vi "LINX - Serial to TCP test.vi"() -> ()   [LabVIEW 2020]
uses:
  <vilib>/MakerHub/LINX/Private/Device/Type Defs/Wifi Config.ctl
  <vilib>/MakerHub/LINX/Private/Type Defs/WIFI Security Type.ctl
  <vilib>/MakerHub/LINX/Private/Device/Type Defs/TCP Config.ctl
  <vilib>/MakerHub/LINX/Public/Utilities/Open Serial.vi
  <vilib>/MakerHub/LINX/Public/Utilities/Open TCP.vi
  <vilib>/MakerHub/LINX/LMH-LINX.lvlib
  <vilib>/MakerHub/LINX/Private/Device/Device.lvlib
panel:
  out "LINX Device Config.TCP Configuration":T1
  in  "stop":bool
  in  "Wifi Configuration":T2={"SSID"="", "IP Address"="0.0.0.0", "Port"=44300, "WIFI Security Type"=enum."WPA2 Password", "Password"=""}
  in  "Serial Port":refnum<visa-resource-name>="N/A"
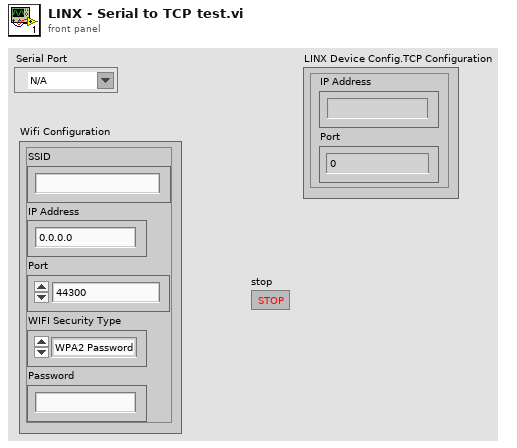
[diagram p1: front panel]
types:
  T1 = typedef "LMH-LINX.lvlib/Device.lvlib/TCP Config.ctl" = cluster{"IP Address":string, "Port":u16}
  T2 = typedef "LMH-LINX.lvlib/Device.lvlib/Wifi Config.ctl" = cluster{"SSID":string, "IP Address":string, "Port":u16, "WIFI Security Type":T3, "Password":string}
  T3 = typedef "LMH-LINX.lvlib/WIFI Security Type.ctl" = enum8{"None", "WPA2 Password", "WPA2 Key", "WEP40", "WEP104"}
  T4 = typedef "LMH-LINX.lvlib/LINX Ref.ctl" = cluster{"IO":T5, "Interface":T6, "LINX Device Config":T7}
  T5 = typedef "LMH-LINX.lvlib/Platform.ctl" = enum16{"Remote", "Local"}
  T6 = typedef "LMH-LINX.lvlib/Interface.ctl" = enum16{"Serial", "TCP"}
  T7 = typedef "LMH-LINX.lvlib/Device.lvlib/LINX Device Config.ctl" = cluster{"Interface":T6, "COM Port":refnum<visa-resource-name>, "TCP Configuration":T1, "Device Family":u8, "Device ID":u8, "Device Name":string, "TCP Ref":refnum<k5>, "Channels":T8}
  T8 = typedef "LMH-LINX.lvlib/Channels.ctl" = cluster{"DI":u8[], "DO":u8[], "AI":u8[], "AO":u8[], "PWM":u8[], "QE":u8[], "UART":u8[], "I2C 2":u8[], "SPI":u8[], "CAN":u8[], "Servo":u8[], "AI Ref (V)":dbl, "AI Resolution (Bits)":u8, "AO Ref (V)":dbl, "AO Resolution (Bits)":u8}
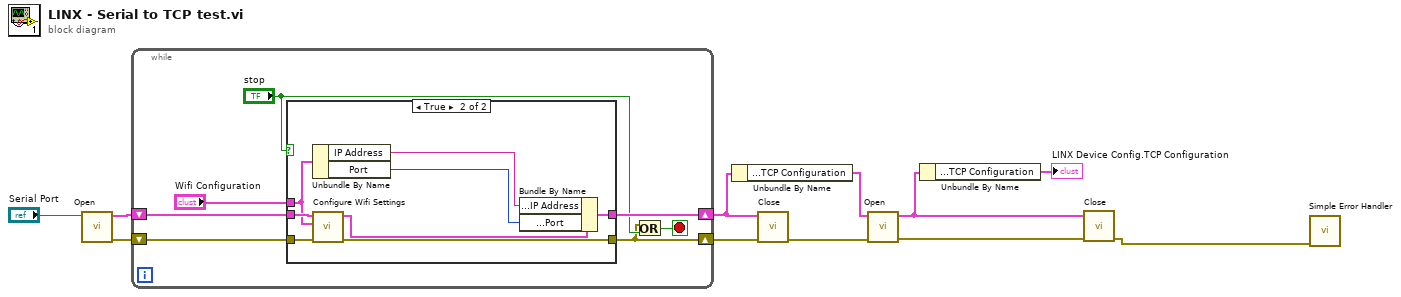
[diagram p0: block diagram]
diagram:
  n1 = call-poly <vilib>:"Open.vi"("Serial Port"="Serial Port") -> ("Error Out"=w10:errorcluster, "LINX Resource"=w9:T4)  [unwired: 8 in, 1 out]
  n2 = while {
    shift-right: [w16] -> w5
    shift-left: w9 -> [w18]
    shift-right: [w13] -> w7
    shift-left: w10 -> [w17]
    stop <- w14 stop-if-true
    n3 = case shown="True" "stop" {
      tunnel: w18 -> [w19 w28]
      tunnel: "Wifi Configuration" -> [_ w24]
      tunnel: w17 -> [w20 w27]
      tunnel: [w19 w23] -> w16
      tunnel: [w20 w25] -> w13
      frame False {
      }
      frame True {
        n4 = Unbundle By Name(w24) -> ("IP Address"=w22:string, "Port"=w21:u16)
        n5 = call <vilib>:"Configure Wifi Settings.vi"("Error In"=w27, "Wifi Configuration"=w24, "LINX Resource"=w28) -> ("Error Out"=w25:errorcluster, "LINX Resource"=w26:T4)  [unwired: 7 in]
        n6 = Bundle By Name(cluster=w26, "LINX Device Config.TCP Configuration.IP Address"=w22, "LINX Device Config.TCP Configuration.Port"=w21) -> (w23:T4)
      }
    }
    n7 = Or(x=w13, y="stop") -> (x .or. y?=w14:bool)
  }
  n8 = Unbundle By Name(w5) -> ("LINX Device Config.TCP Configuration"=w4:T1)
  n9 = call <vilib>:"Close.vi"("Error In"=w7, "LINX Resource"=w5) -> ("Error Out"=w6:errorcluster)  [unwired: 9 in]
  n10 = call-poly <vilib>:"Open.vi"("Error In"=w6, "TCP Configuration"=w4) -> ("Error Out"=w2:errorcluster, "LINX Resource"=w3:T4)  [unwired: 7 in, 1 out]
  n11 = Unbundle By Name(w3) -> ("LINX Device Config.TCP Configuration"=→"LINX Device Config.TCP Configuration":T1)
  n12 = call <vilib>:"Close.vi"("Error In"=w2, "LINX Resource"=w3) -> ("Error Out"=w1:errorcluster)  [unwired: 9 in]
  n13 = call <vilib>:"Simple Error Handler.vi"("error in (no error)"=w1) -> ()  [unwired: 4 in, 5 out]
